vi "Post-Build Action.vi"(5 "Files Generated by Build":path[](array[path]), 6 "Top Level/Always Included VIs":path[](array[path]), 7 "Destination Path":path, 8 "error in (no error)":errorcluster, 9 "Target Name":string, 10 "Build Specification Name":string, 11 "Project Path":path) -> (0 "error out":errorcluster)   [LabVIEW 2020]
uses:
  MeasurementLink Measurement Template/Advanced/MeasurementPlugin.lvclass
  \\10.1.133.57\measurement-services-labview/Source/Measurement Service Template_lv/MeasurementLink Measurement Server/Classes/MeasurementPluginService/MeasurementPluginService.lvclass
  MeasurementLink Measurement Server Internal/RPC Messages/ni_measurementlink_measurement_v1_MeasurementDetails.ctl
  <vilib>/Utility/config.llb/Write Key (String).vi
  <vilib>/ErrorRing/Error Ring.xnode
  <vilib>/Utility/config.llb/NI_LVConfig.lvlib
  MeasurementLink Measurement Server Internal/MeasurementLink Measurement Server Internal.lvlib
  MeasurementLink Measurement Server.lvlib
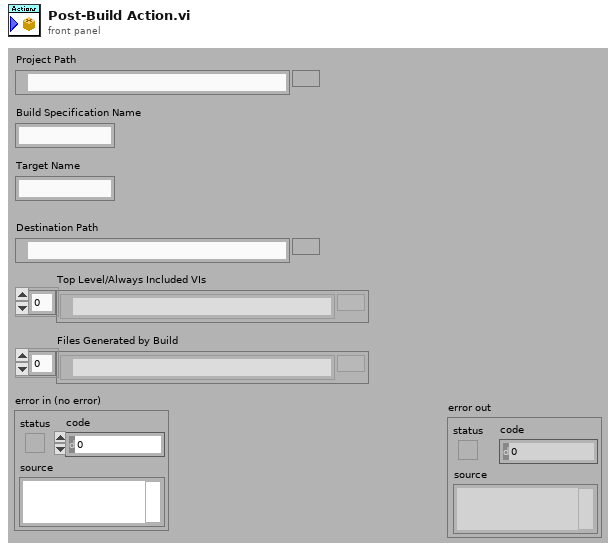
[diagram p1: front panel]
types:
  T1 = cluster{"Target Name":string, "Top Level/Always Included VIs":path[], "Project Path":path, "Destination Path":path, "Build Specification Name":string, "Files Generated by Build":path[]}
  T2 = typedef "MeasurementLink Measurement Server Internal.lvlib/ni_measurementlink_measurement_v1_MeasurementDetails.ctl" = cluster{"display_name":string, "version":string}
  T3 = cluster{"displayName":string, "serviceClass":string, "providedInterfaces":string[], "path":string, "descriptionUrl":string}
  T4 = cluster{"services":cluster{"displayName":string, "serviceClass":string, "providedInterfaces":string[], "path":string, "descriptionUrl":string}[]}
  T5 = typedef "MeasurementLink Measurement Server Internal.lvlib/ni_measurementlink_measurement_v1_UserInterfaceDetails.ctl" = cluster{"file_url":string}
  T6 = cluster{"displayName":string, "serviceClass":string, "providedInterfaces":string[], "path":string, "descriptionUrl":string}[]
  T7 = typedef "NI_LVConfig.lvlib/Config Data RefNum.ctl" = refnum<k1>
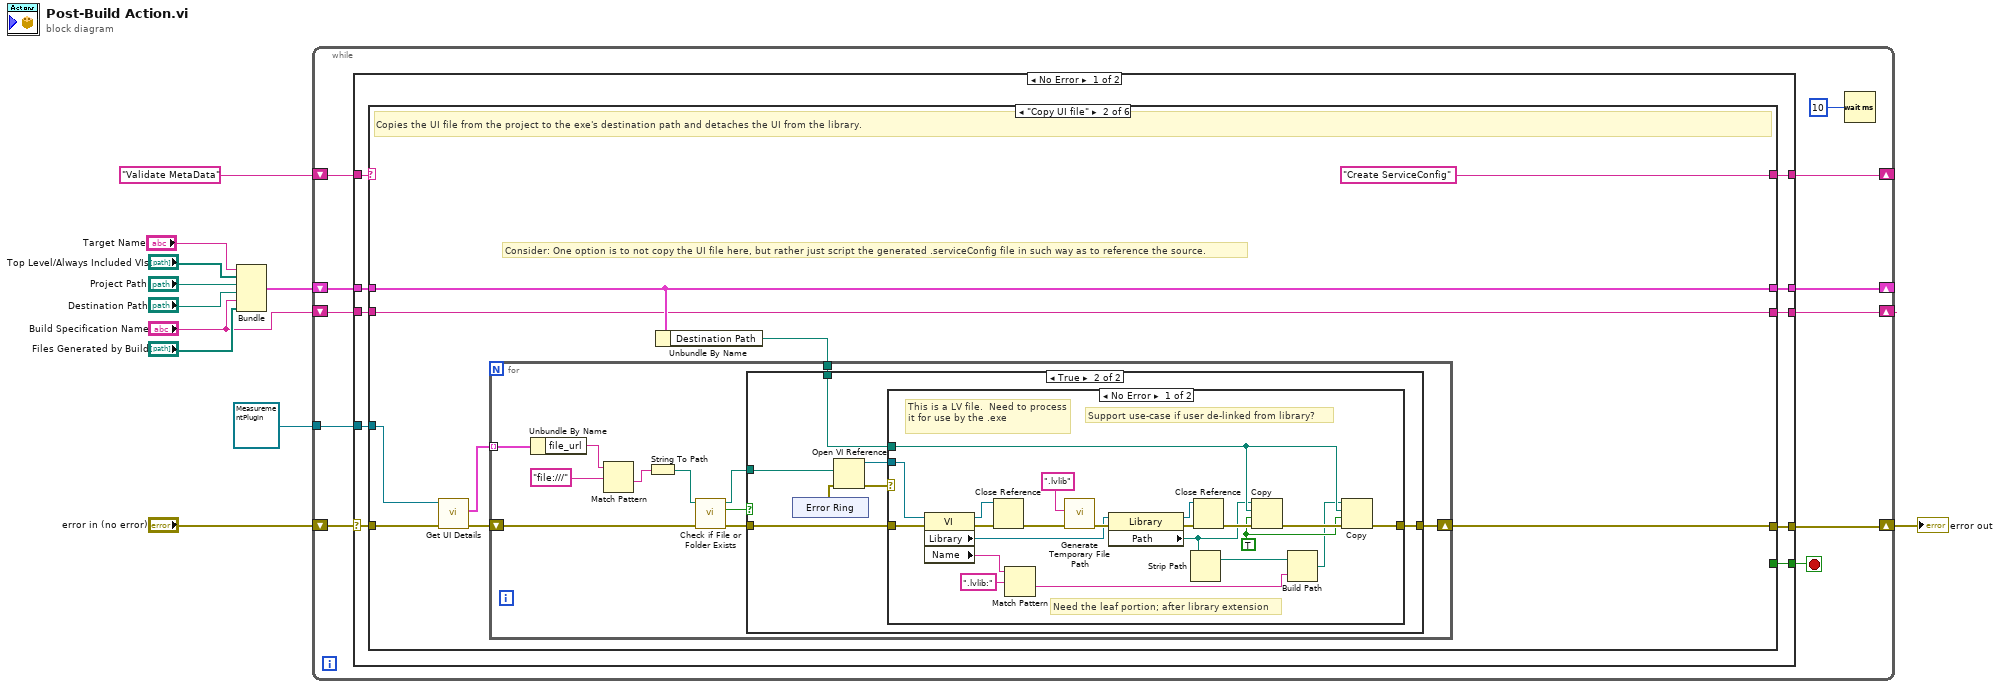
[diagram p0: block diagram]
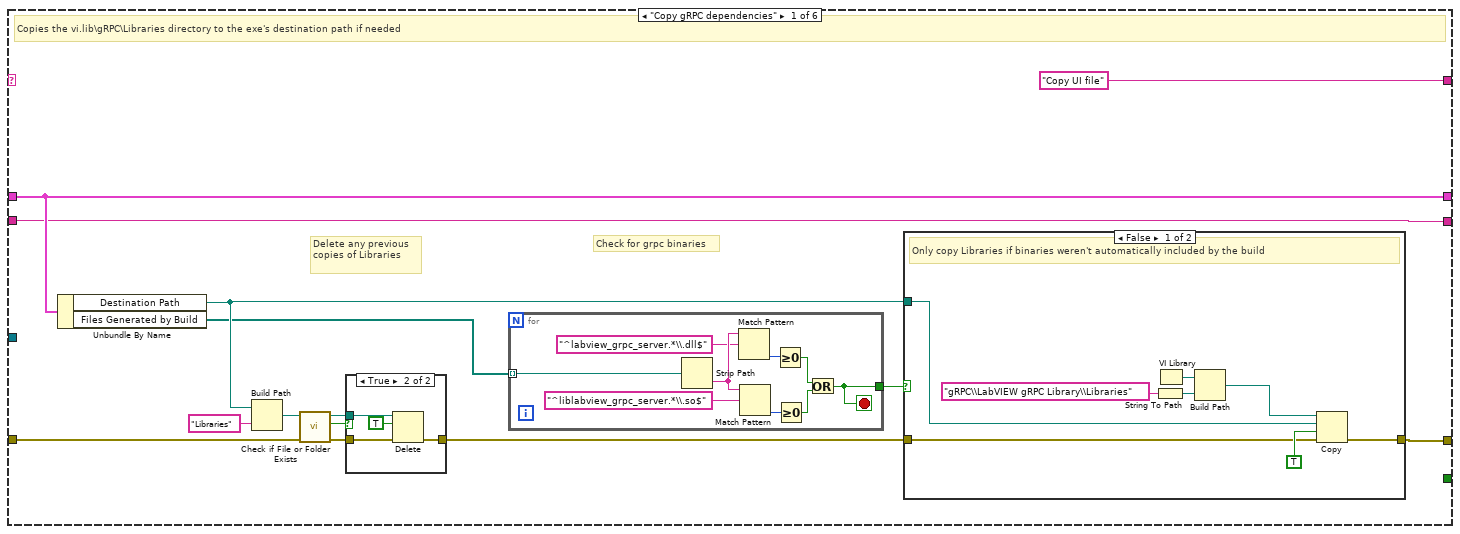
[diagram p2: hidden frame]
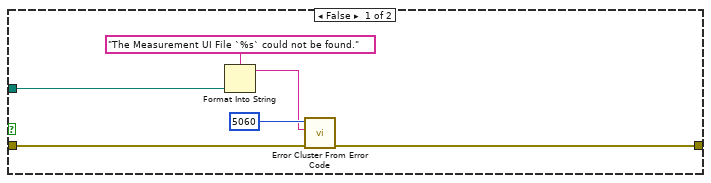
[diagram p5: hidden frame]
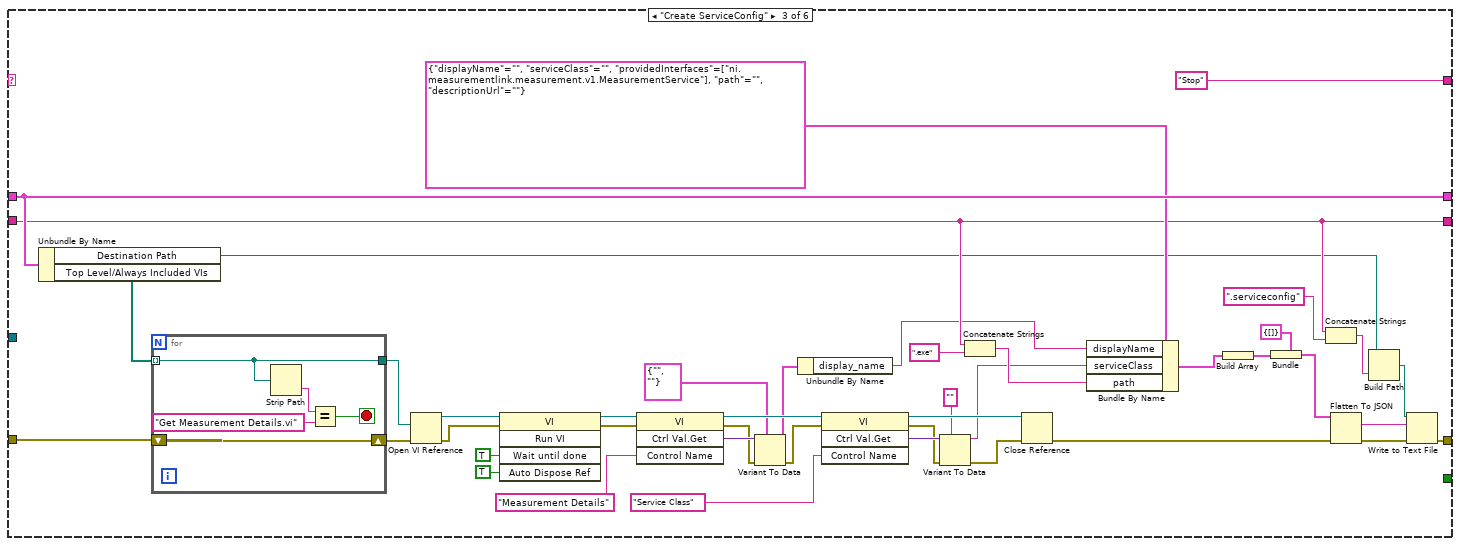
[diagram p7: hidden frame]
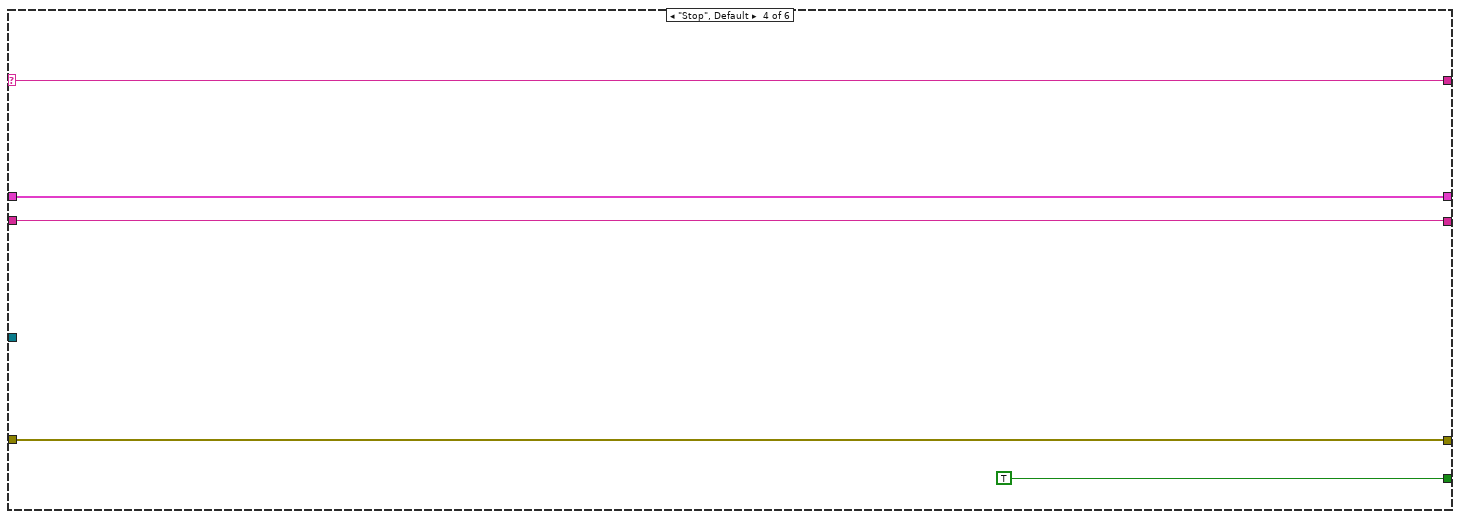
[diagram p8: hidden frame]
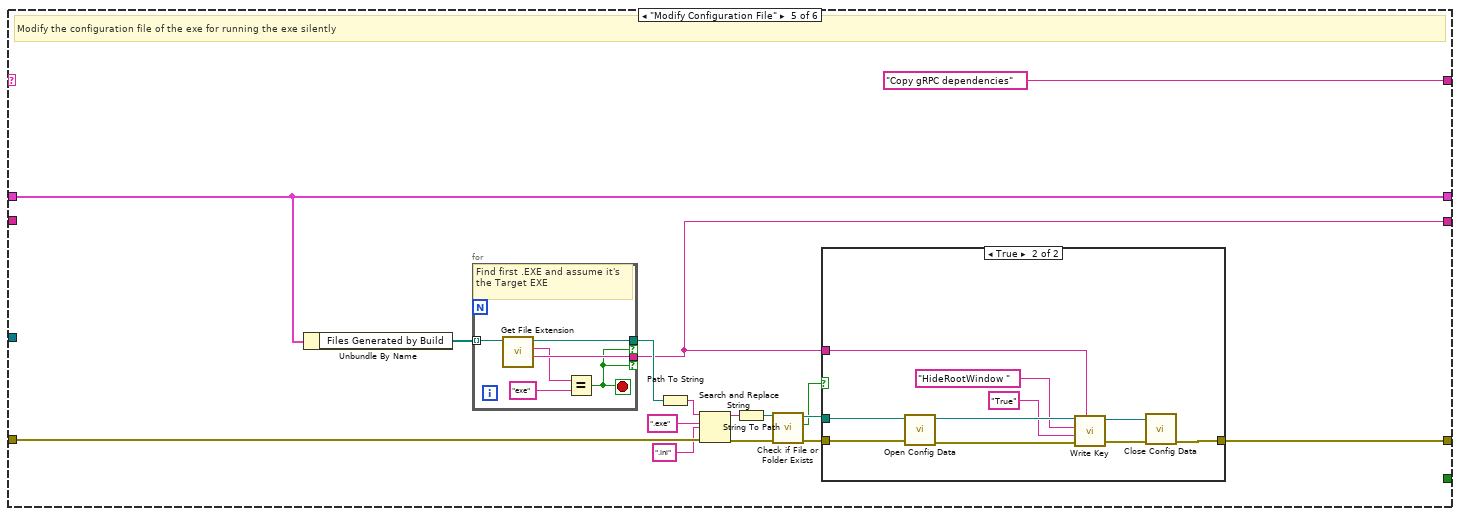
[diagram p9: hidden frame]
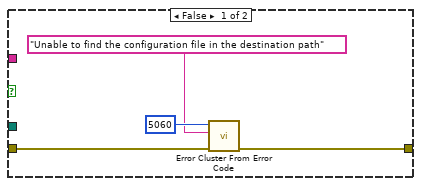
[diagram p10: hidden frame]
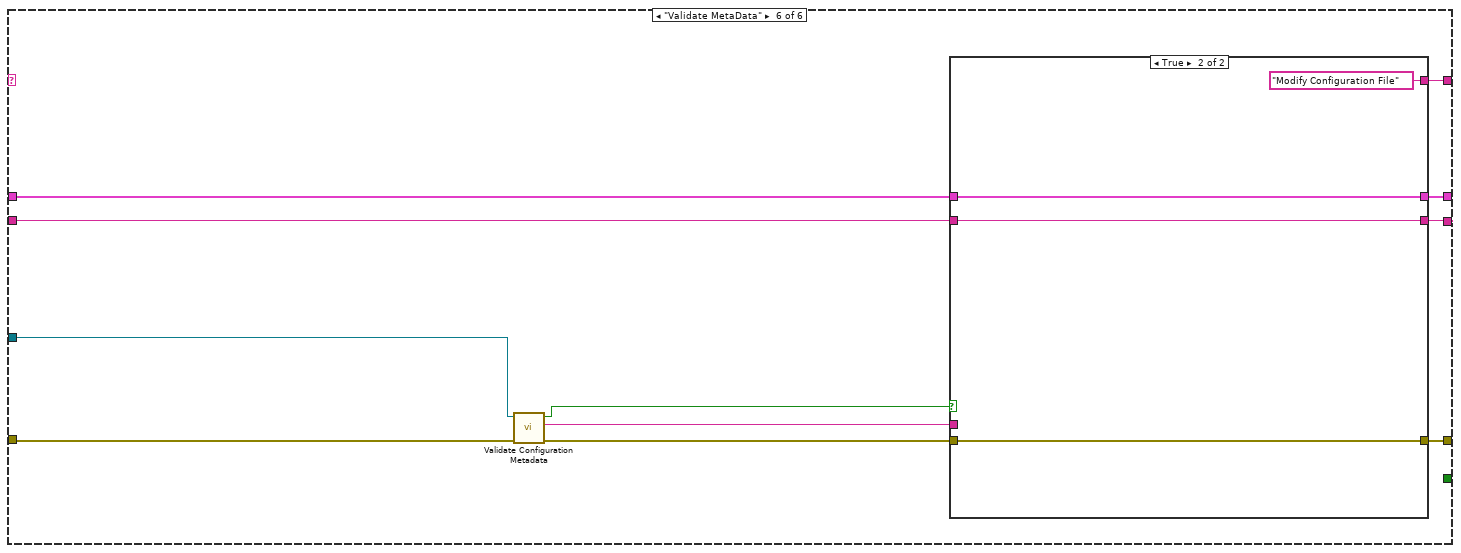
[diagram p11: hidden frame]
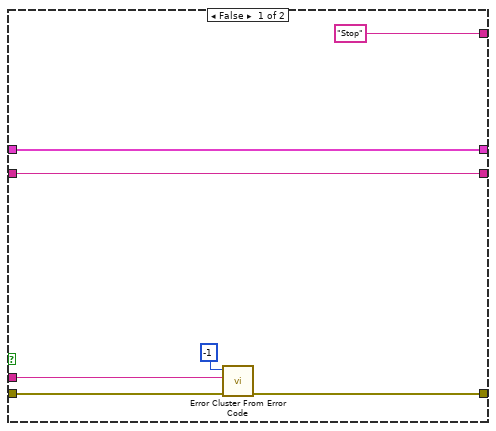
[diagram p12: hidden frame]
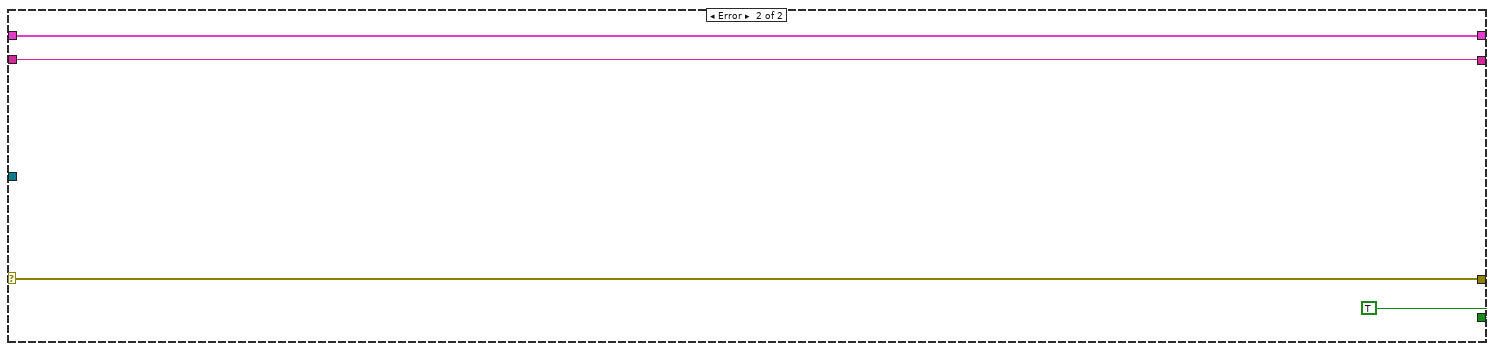
[diagram p13: hidden frame]
diagram:
  n1 = Bundle("Target Name"="Target Name", "Top Level/Always Included VIs"="Top Level/Always Included VIs", "Project Path"="Project Path", "Destination Path"="Destination Path", "Build Specification Name"="Build Specification Name", "Files Generated by Build"="Files Generated by Build") -> (w5:T1)  [unwired: 1 in]
  n2 = while {
    shift-right: [w19] -> _
    shift-left: w5 -> [w20]
    shift-right: [w18] -> w3
    shift-left: "error in (no error)" -> [w15]
    shift-right: [w17] -> _
    shift-left: "Validate MetaData" -> [w21]
    shift-right: [w14] -> _
    shift-left: "Build Specification Name" -> [w13]
    tunnel: refnum<class "MeasurementPlugin.lvclass"> refnum ("MeasurementLink Measurement Template.lvlib:MeasurementPlugin.lvclass") -> [w12]
    stop <- w16 stop-if-true
    n3 = case shown="No Error" w15 {
      selector: w15 -> [w26 w239]
      tunnel: w21 -> [w32 _]
      tunnel: w20 -> [w31 w240]
      tunnel: [w30 w240] -> w19
      tunnel: [w29 w239] -> w18
      tunnel: [w28 _] -> w17
      tunnel: [w27 TRUE] -> w16
      tunnel: [w25 w237] -> w14
      tunnel: w13 -> [w24 w237]
      tunnel: w12 -> [w23 _]
      frame No Error {
        n4 = case shown="\"Copy UI file\"" w32 {
          selector: w32 -> [_ _ _ w176 _ _]
          tunnel: w31 -> [w44 w78 w167 w178 w190 w224]
          tunnel: [w44 w78 w167 w178 w190 w223] -> w30
          tunnel: w26 -> [w36 w73 w166 w175 w188 w219]
          tunnel: [w46 w77 w131 w175 w194 w225] -> w29
          tunnel: ["Copy UI file" "Create ServiceConfig" "Stop" w176 "Copy gRPC dependencies" w220] -> w28
          tunnel: [_ _ _ TRUE _ _] -> w27
          tunnel: [w43 w74 w137 w174 w180 w221] -> w25
          tunnel: w24 -> [w43 w74 w137 w174 _ w222]
          tunnel: w23 -> [_ w72 _ _ _ w218]
          frame "Copy gRPC dependencies" {
            # "Delete any previous copies of Libraries"
            # "Check for grpc binaries"
            # "Copies the vi.lib\\gRPC\\Libraries directory to the exe's destination path if needed"
            n5 = Unbundle By Name(w44) -> ("Destination Path"=w35:path, "Files Generated by Build"=w33:path[])
            n6 = Build Path(base path=w35, name or relative path="Libraries") -> (appended path=w41:path)
            n7 = call <vilib>:"Check if File or Folder Exists.vi"("error in (no error)"=w36, "path"=w41) -> ("error out"=w40:errorcluster, "file or folder exists?"=w38:bool, "dup path"=w39:path)  [unwired: 7 in]
            n8 = case shown="True" w38 {
              tunnel: w40 -> [w56 w60]
              tunnel: [w56 w59] -> w34
              tunnel: w39 -> [_ w57]
              frame False {
              }
              frame True {
                n9 = Delete(path (use dialog)=w57, entire hierarchy (F)=TRUE ("confirm (F)"), error in=w60) -> (error out=w59:errorcluster)  [unwired: 2 in, 2 out]
              }
            }
            n10 = for {
              tunnel: [w47] -> w42
              tunnel: w33 -> [w52] mode=indexing
              stop <- w47 stop-if-true
              n11 = Strip Path(path=w52) -> (name=w55:string)  [unwired: 1 out]
              n12 = Match Pattern(string=w55, regular expression="^labview_grpc_server.*\\.dll$" ("pattern")) -> (offset past match=w51:i32)  [unwired: 1 in, 3 out]
              n13 = Match Pattern(string=w55, regular expression="^liblabview_grpc_server.*\\.so$" ("pattern")) -> (offset past match=w50:i32)  [unwired: 1 in, 3 out]
              n14 = Greater Or Equal To 0?(x=w51) -> (x >= 0?=w49:bool)
              n15 = Greater Or Equal To 0?(x=w50) -> (x >= 0?=w48:bool)
              n16 = Or(x=w49, y=w48) -> (x .or. y?=w47:bool)
            }
            n17 = case shown="False" w42 {
              tunnel: [w64 w69] -> w46
              tunnel: w35 -> [w62 _]
              tunnel: w34 -> [w61 w69]
              frame False {
                # "Only copy Libraries if binaries weren't automatically included by the build"
                n18 = String To Path(string="gRPC\\LabVIEW gRPC Library\\Libraries") -> (path=w66:path)
                n19 = VI Library() -> (path=w68:path)
                n20 = Build Path(base path=w68, name or relative path=w66) -> (appended path=w65:path)
                n21 = Copy(8:w61, 9:TRUE ("overwrite (F)"), 10:w62, 11:w65) -> (0:w64:errorcluster)  [unwired: 1 in, 2 out]
              }
              frame True {
              }
            }
          }
          frame "Copy UI file" {
            # "Consider: One option is to not copy the UI file here, but rather just script the generated .serviceConfig file in such way as to reference the source."
            # "Copies the UI file from the project to the exe's destination path and detaches the UI from the library."
            n22 = call-dynamic "Get UI Details.vi"("error in"=w73, "gRPC Server in"=w72) -> ("error out"=w71:errorcluster, "user_interface_details"=w70:T5[])  [unwired: 7 in, 1 out]
            n23 = Unbundle By Name(w78) -> ("Destination Path"=w75:path)
            n24 = for {
              tunnel: w75 -> [w84]
              tunnel: w70 -> [w88] mode=indexing
              shift-right: [w89] -> w77
              shift-left: w71 -> [w83]
              n25 = Unbundle By Name(w88) -> ("file_url"=w86:string)
              n26 = Match Pattern(string=w86, regular expression="file:///") -> (after substring=w85:string)  [unwired: 1 in, 3 out]
              n27 = String To Path(string=w85) -> (path=w81:path)
              n28 = call <vilib>:"Check if File or Folder Exists.vi"("error in (no error)"=w83, "path"=w81) -> ("error out"=w82:errorcluster, "file or folder exists?"=w79:bool, "dup path"=w80:path)  [unwired: 7 in]
              n29 = case shown="True" w79 {
                tunnel: [w93 w102] -> w89
                tunnel: w84 -> [_ w98]
                tunnel: w82 -> [w94 w97]
                tunnel: w80 -> [w91 w96]
                frame False {
                  n30 = Format Into String(format string="The Measurement UI File `%s` could not be found." ("error message (\"\")"), w91) -> (resulting string=w90:string)  [unwired: 2 in, 1 out]
                  n31 = call <vilib>:"Error Cluster From Error Code.vi"("error in (no error)"=w94, "error message (\"\")"=w90, "error code (0)"=5060) -> ("error out"=w93:errorcluster)  [unwired: 6 in]
                }
                frame True {
                  n32 = xnode "Error Ring"() -> ("error out"=w101:errorcluster)
                  n33 = Open VI Reference(vi path=w96, error in (no error)=w101) -> (vi reference=w99:refnum<vi>, error out=w100:errorcluster)  [unwired: 4 in]
                  n34 = case shown="No Error" w100 {
                    tunnel: w97 -> [w123 w125]
                    tunnel: [w104 w125] -> w102
                    tunnel: w99 -> [w124 _]
                    tunnel: w98 -> [w109 _]
                    frame No Error {
                      w110 = TRUE ("overwrite (F)")
                      # "Support use-case if user de-linked from library?"
                      # "Need the leaf portion; after library extension"
                      # "This is a LV file.  Need to process it for use by the .exe"
                      n35 = property class="VI"(reference=w124, error in=w123) -> (reference out=w121:refnum<vi>, error out=w120:errorcluster, "Library"=w115:refnum<vi>, "Name"=w118:string)
                      n36 = Close Reference(reference=w121, error in (no error)=w120) -> (error out=w119:errorcluster)
                      n37 = Match Pattern(string=w118, regular expression=".lvlib:") -> (after substring=w106:string)  [unwired: 1 in, 3 out]
                      n38 = call <vilib>:"Generate Temporary File Path.vi"("error in (no error)"=w119, "Temporary File Extension (tmp)"=".lvlib") -> ("error out"=w116:errorcluster)  [unwired: 8 in, 1 out]
                      n39 = property class="Library"(reference=w115, error in=w116) -> (reference out=w114:refnum<vi>, error out=w113:errorcluster, "Path"=w108:path)
                      n40 = Strip Path(path=w108) -> (stripped path=w107:path)  [unwired: 1 out]
                      n41 = Close Reference(reference=w114, error in (no error)=w113) -> (error out=w112:errorcluster)
                      n42 = Copy(8:w112, 9:w110, 10:w109, 11:w108) -> (0:w111:errorcluster)  [unwired: 1 in, 2 out]
                      n43 = Build Path(base path=w107, name or relative path=w106) -> (appended path=w105:path)
                      n44 = Copy(8:w111, 9:w110, 10:w109, 11:w105) -> (0:w104:errorcluster)  [unwired: 1 in, 2 out]
                    }
                    frame Error {
                      # "This is not a LV file.  No need to process it or make a copy."
                    }
                  }
                }
              }
            }
          }
          frame "Create ServiceConfig" {
            n45 = Unbundle By Name(w167) -> ("Destination Path"=w135:path, "Top Level/Always Included VIs"=w168:path[])
            n46 = for {
              tunnel: w168 -> [w171] mode=indexing
              tunnel: [w171] -> w165
              shift-right: [w169] -> w164
              shift-left: w166 -> [w169]
              stop <- w172 stop-if-true
              n47 = Strip Path(path=w171) -> (name=w173:string)  [unwired: 1 out]
              n48 = Equal?(x=w173, y="Get Measurement Details.vi") -> (x = y?=w172:bool)
            }
            n49 = Open VI Reference(vi path=w165, error in (no error)=w164) -> (vi reference=w163:refnum<vi>, error out=w155:errorcluster)  [unwired: 4 in]
            n50 = invoke class="VI" method="Run VI"(reference=w163, error in=w155, "Wait until done"=TRUE ("Wait Until Done"), "Auto Dispose Ref"=TRUE ("Auto Dispose Reference")) -> (reference out=w160:refnum<vi>, error out=w156:errorcluster)  [unwired: 1 in, 3 out]
            n51 = invoke class="VI" method="Ctrl Val.Get"(reference=w160, error in=w156, "Control Name"="Measurement Details") -> (reference out=w157:refnum<vi>, error out=w151:errorcluster, "Get Control Value Variant"=w152:variant)  [unwired: 1 in, 1 out]
            n52 = Variant To Data(error in=w151, type=T2 {"display_name"="", "version"=""} ("ni_measurements_v1_MeasurementDetails"), Variant=w152) -> (data=w140:T2, error out=w150:errorcluster)
            n53 = Unbundle By Name(w140) -> ("display_name"=w127:string)
            n54 = invoke class="VI" method="Ctrl Val.Get"(reference=w157, error in=w150, "Control Name"="Service Class") -> (reference out=w154:refnum<vi>, error out=w148:errorcluster, "Get Control Value Variant"=w149:variant)  [unwired: 1 in, 1 out]
            n55 = Variant To Data(error in=w148, type="", Variant=w149) -> (data=w126:string, error out=w147:errorcluster)
            n56 = Concatenate Strings(w137, ".exe" ("string")) -> (w128:string)
            n57 = Close Reference(reference=w154, error in (no error)=w147) -> (error out=w133:errorcluster)
            n58 = Bundle By Name(cluster=T3 {"displayName"="", "serviceClass"="", "providedInterfaces"=["ni.measurementlink.measurement.v1.MeasurementService"], "path"="", "descriptionUrl"=""}, "displayName"=w127, "serviceClass"=w126, "path"=w128) -> (w142:T3)
            n59 = Build Array(w142) -> (w141:T6)
            n60 = Bundle(cluster=T4 {"services"=[]}, "services"=w141) -> (w139:T4)
            n61 = Concatenate Strings(w137, ".serviceconfig" ("string")) -> (w134:string)
            n62 = Flatten To JSON(anything=w139, error in (no error)=w133) -> (JSON string=w138:string, 11:w132:errorcluster)  [unwired: 1 in]
            n63 = Build Path(base path=w135, name or relative path=w134) -> (appended path=w130:path)
            n64 = Write to Text File(file (use dialog)=w130, text=w138, error in=w132) -> (error out=w131:errorcluster)  [unwired: 1 in, 2 out]
          }
          frame "Stop", Default {
          }
          frame "Modify Configuration File" {
            # "Modify the configuration file of the exe for running the exe silently"
            n65 = Unbundle By Name(w190) -> ("Files Generated by Build"=w189:path[])
            n66 = for {
              tunnel: w189 -> [w200] mode=indexing
              tunnel: [w199] -> w180 if=w195
              tunnel: [w198] -> w182 if=w195
              stop <- w195 stop-if-true
              # "Find first .EXE and assume it's the Target EXE"
              n67 = call <vilib>:"Get File Extension.vi"("file"=w200) -> ("filename without extension"=w199:string, "lowercase file extension"=w196:string, "dup file"=w198:path)  [unwired: 6 in, 2 out]
              n68 = Equal?(x=w196, y="exe") -> (x = y?=w195:bool)
            }
            n69 = Path To String(path=w182) -> (string=w181:string)
            n70 = Search and Replace String(input string=w181, search string=".exe", replace string=".ini", error in=w188) -> (result string=w185:string, error out=w187:errorcluster)  [unwired: 4 in, 2 out]
            n71 = String To Path(string=w185) -> (path=w184:path)
            n72 = call <vilib>:"Check if File or Folder Exists.vi"("error in (no error)"=w187, "path"=w184) -> ("error out"=w193:errorcluster, "file or folder exists?"=w191:bool, "dup path"=w192:path)  [unwired: 7 in]
            n73 = case shown="True" w191 {
              tunnel: [w203 w214] -> w194
              tunnel: w192 -> [_ w207]
              tunnel: w193 -> [w204 w206]
              tunnel: w180 -> [_ w205]
              frame False {
                n74 = call <vilib>:"Error Cluster From Error Code.vi"("error in (no error)"=w204, "error message (\"\")"="Unable to find the configuration file in the destination path" ("source"), "error code (0)"=5060) -> ("error out"=w203:errorcluster)  [unwired: 6 in]
              }
              frame True {
                n75 = call <vilib>:"Open Config Data.vi"("error in (no error)"=w206, "configuration file path"=w207) -> ("error out"=w213:errorcluster, "refnum"=w212:T7)  [unwired: 7 in, 1 out]
                n76 = call-poly <vilib>:"Write Key.vi"("section"=w205, "error in (no error)"=w213, "value"="True", "key"="HideRootWindow ", "refnum"=w212) -> ("error out"=w210:errorcluster, "refnum out"=w209:T7)  [unwired: 4 in, 1 out]
                n77 = call <vilib>:"Close Config Data.vi"("error in (no error)"=w210, "refnum"=w209) -> ("error out"=w214:errorcluster)  [unwired: 8 in, 1 out]
              }
            }
          }
          frame "Validate MetaData" {
            n78 = call "Validate Configuration Metadata.vi"("error in (no error)"=w219, "Measurement"=w218) -> ("error out"=w215:errorcluster, "Invalid Parameters"=w216:string, "Is Metadata Valid"=w217:bool)  [unwired: 7 in]
            n79 = case shown="True" w217 {
              tunnel: w215 -> [w229 w236]
              tunnel: [w228 w236] -> w225
              tunnel: w216 -> [w226 _]
              tunnel: w224 -> [w232 w235]
              tunnel: [w232 w235] -> w223
              tunnel: w222 -> [w231 w234]
              tunnel: [w231 w234] -> w221
              tunnel: ["Stop" "Modify Configuration File"] -> w220
              frame False {
                n80 = call <vilib>:"Error Cluster From Error Code.vi"("error in (no error)"=w229, "error message (\"\")"=w226, "error code (0)"=-1) -> ("error out"=w228:errorcluster)  [unwired: 6 in]
              }
              frame True {
              }
            }
          }
        }
      }
      frame Error {
      }
    }
    n81 = Wait (ms)(milliseconds to wait=u32 10 ("millisecond timer value")) -> ()  [unwired: 1 out]
  }
  "error out" <- w3
